vi "Subscriber-TCSS.vi"() -> (3 "OSS_Supervisory":T1)   [LabVIEW 2019]
uses:
  OSS_Supervisory.ctl
  <vilib>/Distrio/LabbitMQ/Channel/exchange_type_enum.ctl
  <vilib>/Distrio/LabbitMQ/Connection/Connection.lvclass
  <vilib>/Distrio/LabbitMQ/Connection/connection_parameters_cluster.ctl
  <vilib>/Distrio/LabbitMQ/Channel/Channel.lvclass
  <vilib>/Distrio/LabbitMQ/Queue/Queue.lvclass
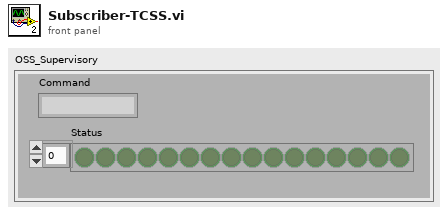
[diagram p1: front panel]
types:
  T1 = typedef "OSS_Supervisory.ctl" = cluster{"Command":string, "Status":bool[]}
  T2 = typedef "Connection.lvclass/connection_parameters_cluster.ctl" = cluster{"host name":string, "port":i32, "user name":string, "password":string, "virtual host":string}
  T3 = typedef "Channel.lvclass/exchange_type_enum.ctl" = enum16{"direct", "topic", "fanout", "headers"}
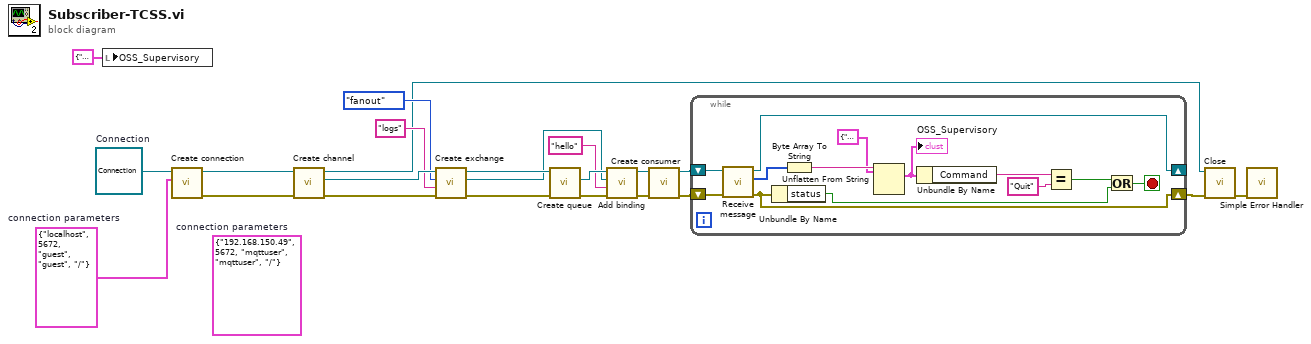
[diagram p0: block diagram]
diagram:
  (unwired) T2 {"host name"="192.168.150.49", "port"=5672, "user name"="mqttuser", "password"="mqttuser", "virtual host"="/"}  # connection parameters
  w7 = T2 {"host name"="localhost", "port"=5672, "user name"="guest", "password"="guest", "virtual host"="/"}  # connection parameters
  w8 = refnum<class "Connection.lvclass"> refnum  # Connection
  n1 = local write "OSS_Supervisory"(cluster{"Command":string, "Status":bool[]} {"Command"="", "Status"=[FALSE]} ("OSS_Supervisory")) -> ()
  n2 = call <vilib>:"Create connection.vi"("connection parameters"=w7, "Connection in"=w8) -> ("error out"=w21:errorcluster, "Connection out"=w22:refnum<class "Connection.lvclass">)  [unwired: 8 in]
  n3 = call <vilib>:"Create channel.vi"("error in (no error)"=w21, "Connection in"=w22) -> ("error out"=w20:errorcluster, "channel"=w19:refnum<class "Channel.lvclass">, "Connection out"=w6:refnum<class "Connection.lvclass">)  [unwired: 7 in]
  n4 = call <vilib>:"Create exchange.vi"("error in (no error)"=w20, "exchange name"="logs", "exchange type"=exchange_type_enum."fanout" ("binding"), "Channel in"=w19) -> ("error out"=w18:errorcluster, "Exchange.lvclass"=w14:refnum<class "Exchange.lvclass">, "Channel out"=w17:refnum<class "Channel.lvclass">)  [unwired: 5 in]
  n5 = call <vilib>:"Create queue.vi"("error in (no error)"=w18, "Channel in"=w17) -> ("error out"=w16:errorcluster, "Queue.lvclass"=w15:refnum<class "Queue.lvclass">)  [unwired: 7 in, 1 out]
  n6 = call <vilib>:"Add binding.vi"("error in (no error)"=w16, "binding key"="hello" ("routing key"), "Exchange.lvclass"=w14, "Consumer in"=w15) -> ("error out"=w12:errorcluster, "Consumer out"=w11:refnum<class "Queue.lvclass">)  [unwired: 6 in]
  n7 = call <vilib>:"Create consumer.vi"("error in (no error)"=w12, "Queue in"=w11) -> ("error out"=w3:errorcluster, "Queue out"=w4:refnum<class "Queue.lvclass">)  [unwired: 8 in]
  n8 = while {
    shift-right: [w32] -> _
    shift-left: w4 -> [w34]
    shift-right: [w31] -> w2
    shift-left: w3 -> [w33]
    stop <- w25 stop-if-true
    n9 = call <vilib>:"Receive message.vi"("error in (no error)"=w33, "Consumer in"=w34) -> ("error out"=w31:errorcluster, "message body"=w35:u8[], "Consumer out"=w32:refnum<class "Queue.lvclass">)  [unwired: 4 in, 3 out]
    n10 = Unbundle By Name(w31) -> ("status"=w23:bool)
    n11 = Byte Array To String(unsigned byte array=w35) -> (string=w30:string)
    n12 = Unflatten From String(type=cluster{"Command":string, "Status":bool[]} {"Command"="", "Status"=[FALSE]} ("OSS_Supervisory"), binary string=w30) -> (value=w27:cluster{"Command":string, "Status":bool[]})  [unwired: 3 in, 2 out]
    "OSS_Supervisory" <- w27
    n13 = Unbundle By Name(w27) -> ("Command"=w28:string)
    n14 = Equal?(x=w28, y="Quit") -> (x = y?=w24:bool)
    n15 = Or(x=w24, y=w23) -> (x .or. y?=w25:bool)
  }
  n16 = call <vilib>:"Close.vi"("error in (no error)"=w2, "Connection in"=w6) -> ("error out"=w5:errorcluster)  [unwired: 8 in, 1 out]
  n17 = call <vilib>:"Simple Error Handler.vi"("error in (no error)"=w5) -> ()  [unwired: 4 in, 5 out]
